vi "Execute.vi"(8 "error in (no error)":errorcluster, 10 "Execution":refnum<data-value>, 11 "StepBase in":refnum<class "Step.lvclass">) -> (0 "error out":errorcluster, 1 "Output Values":cluster{"Name":string, "Variant Data":variant}[](array[cluster]), 3 "StepBase out":refnum<class "Step.lvclass">)   [LabVIEW 2015, in "Step.lvclass"]
uses:
  Step.lvclass
  Execution.lvclass
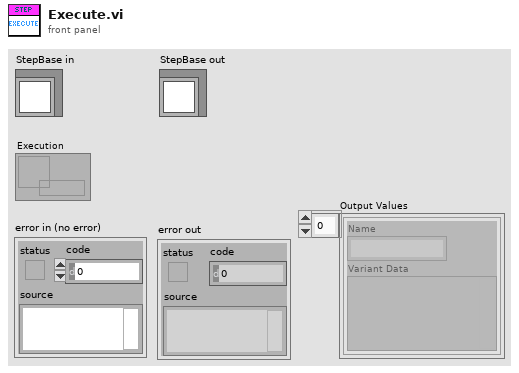
[diagram p1: front panel]
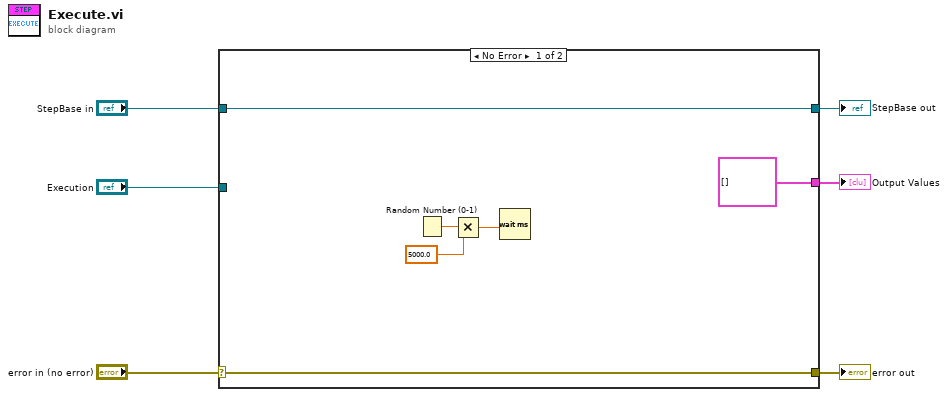
[diagram p0: block diagram]
diagram:
  n1 = case shown="No Error" "error in (no error)" {
    selector: "error in (no error)" -> [w12 w14]
    tunnel: [w12 w14] -> w5
    tunnel: [w11 w13] -> w3
    tunnel: "StepBase in" -> [w11 w13]
    tunnel: [cluster{"Name":string, "Variant Data":variant}[] [] ("Output Values") _] -> w2
    tunnel: "Execution" -> [_ _]
    frame No Error {
      n2 = Random Number (0-1)() -> (number: 0 to 1=w10:dbl)
      n3 = Multiply(x=w10, y=5000.0) -> (x*y=w9:dbl)
      n4 = Wait (ms)(milliseconds to wait=w9) -> ()  [unwired: 1 out]
    }
    frame Error {
    }
  }
  "error out" <- w5
  "StepBase out" <- w3
  "Output Values" <- w2
